vi "IOC shared memory de-initialize.vi"(0 "shared memory in":T1, 3 "error in (no error)":errorcluster) -> ()   [LabVIEW 2017, in "linuxSharedMemory.lvlib"]
uses:
  linuxSharedMemory.lvlib
  <vilib>/NI/NI Linux RT IPC/Shared Memory/Controls/reference.ctl
  <vilib>/NI/NI Linux RT IPC/Shared Memory/Classes/Shared Memory/Shared Memory.lvclass
  <vilib>/NI/NI Linux RT IPC/Shared Memory/Linux RT IPC.Shared Memory.lvlib
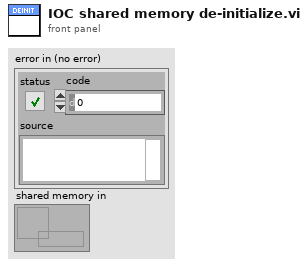
[diagram p1: front panel]
types:
  T1 = typedef "Linux RT IPC.Shared Memory.lvlib/reference.ctl" = refnum<data-value>
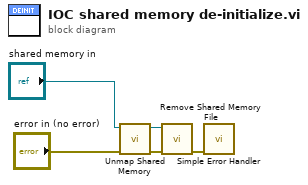
[diagram p0: block diagram]
diagram:
  n1 = call <vilib>:"Unmap Shared Memory.vi"("error in (no error)"="error in (no error)", "shared memory in"="shared memory in") -> ("error out"=w4:errorcluster, "shared memory out"=w3:T1)  [unwired: 8 in]
  n2 = call <vilib>:"Remove Shared Memory File.vi"("error in (no error)"=w4, "shared memory in"=w3) -> ("error out"=w5:errorcluster)  [unwired: 8 in, 1 out]
  n3 = call <vilib>:"Simple Error Handler.vi"("error in (no error)"=w5) -> ()  [unwired: 4 in, 5 out]
